vi "Unflatten Packet Header.vi"(8 "error in (no error)":errorcluster, 10 "Bytes in":u8[](array[numeric]), 11 "pcap Parse and Build in":refnum<class "pcap Parse and Build.lvclass">) -> (0 "error out":errorcluster, 1 "Packet Header":T1, 2 "Bytes out":u8[](array[numeric]), 3 "pcap Parse and Build out":refnum<class "pcap Parse and Build.lvclass">)   [LabVIEW 2021, in "pcap Parse and Build.lvclass"]
uses:
  pcap Parse and Build.lvclass
  Typedef/Packet Header.ctl
  pcap Parse and Build.lvclass/pcap Parse and Build.ctl
  Typedef/Errors.ctl
  a43927ee-7cb0-4c47-8c72-c2f3daaaf6fd.vi
  a43927ee-7cb0-4c47-8c72-c2f3daaaf6fd.vi/c28b0ead-42ad-4072-80a2-aca7f2bd7ce3.vi
  <vilib>/CIF Foundation/CIF Utilities/Errors/Append Error Location.vi
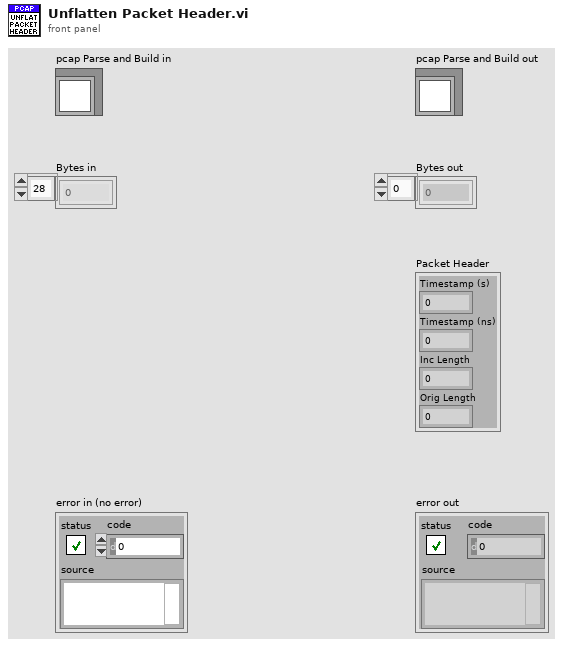
[diagram p1: front panel]
types:
  T1 = typedef "pcap Parse and Build.lvclass/Packet Header.ctl" = cluster{"Timestamp (s)":u32, "Timestamp (ns)":u32, "Inc Length":u32, "Orig Length":u32}
  T2 = typedef "pcap Parse and Build.lvclass/Errors.ctl" = enum16{"Invalid Global Header", "Out of Data"}
  T3 = typedef "pcap Parse and Build.lvclass/Time Format.ctl" = enum16{"us", "ns"}
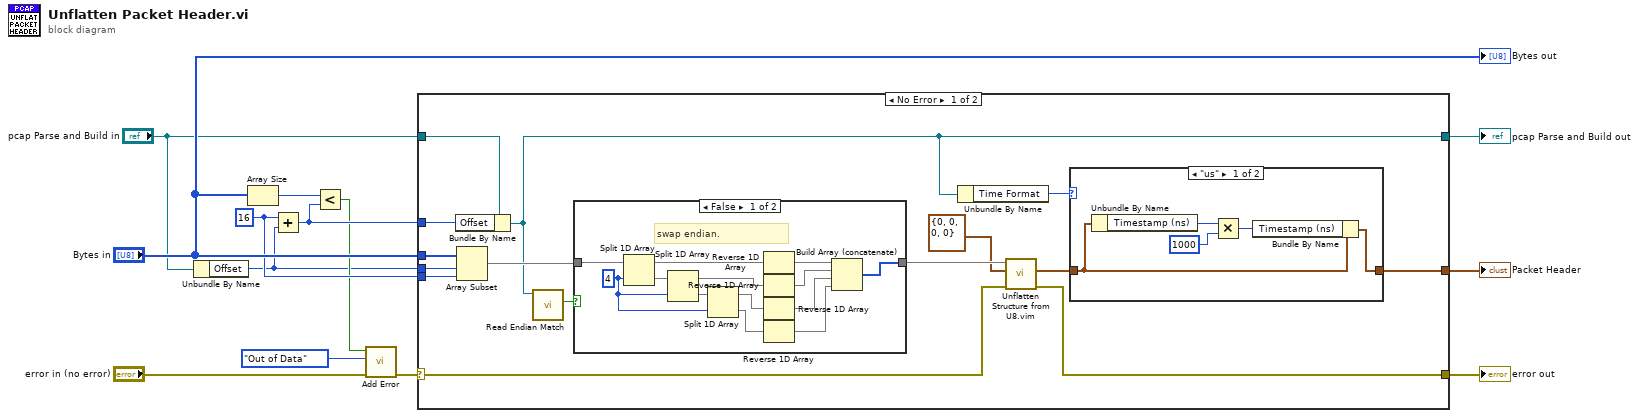
[diagram p0: block diagram]
diagram:
  w10 = 16 ("length")
  n1 = Unbundle By Name("pcap Parse and Build in") -> ("Offset"=w3:i32)
  n2 = Array Size(array="Bytes in") -> (size(s)=w5:i32)
  n3 = Add(x=w10, y=w3) -> (x+y=w11:i32)
  n4 = Less?(x=w5, y=w11) -> (x < y?=w9:bool)
  n5 = call "Add Error.vi"("error in (no error)"="error in (no error)", "Error"=Errors."Out of Data", "Insert Error"=w9) -> ("error out"=w6:errorcluster)  [unwired: 8 in]
  n6 = case shown="No Error" w6 {
    selector: w6 -> [w27 w50]
    tunnel: [w28 w50] -> w4
    tunnel: [w23 _] -> w13
    tunnel: "Bytes in" -> [w25 _]
    tunnel: w11 -> [w19 _]
    tunnel: w10 -> [w22 _]
    tunnel: w3 -> [w21 _]
    tunnel: "pcap Parse and Build in" -> [w20 w49]
    tunnel: [w17 w49] -> w1
    frame No Error {
      n7 = Bundle By Name(cluster=w20, "Offset"=w19) -> (w17:refnum<class "pcap Parse and Build.lvclass">)
      n8 = Array Subset(array=w25, index=w21, length=w22) -> (w24:u8[])
      n9 = call "Read Endian Match.vi"("pcap Parse and Build in"=w17) -> ("Endian Match"=w18:bool)  [unwired: 8 in, 2 out]
      n10 = case shown="False" w18 {
        tunnel: w24 -> [w34 w42]
        tunnel: [w29 w42] -> w26
        frame False {
          w39 = 4 ("index")
          # "swap endian."
          n11 = Split 1D Array(array=w34, index=w39) -> (first subarray=w37:u8[], second subarray=w41:u8[])
          n12 = Split 1D Array(array=w41, index=w39) -> (first subarray=w36:u8[], second subarray=w40:u8[])
          n13 = Split 1D Array(array=w40, index=w39) -> (first subarray=w35:u8[], second subarray=w38:u8[])
          n14 = Reverse 1D Array(array=w37) -> (reversed array=w33:u8[])
          n15 = Reverse 1D Array(array=w36) -> (reversed array=w32:u8[])
          n16 = Reverse 1D Array(array=w35) -> (reversed array=w31:u8[])
          n17 = Reverse 1D Array(array=w38) -> (reversed array=w30:u8[])
          n18 = Build Array (concatenate)(w33, w32, w31, w30) -> (w29:u8[])
        }
        frame True {
        }
      }
      n19 = Unbundle By Name(w17) -> ("Time Format"=w16:T3)
      n20 = call "Unflatten Structure from U8.vim"("error in"=w27, "Type"=T1 {"Timestamp (s)"=0, "Timestamp (ns)"=0, "Inc Length"=0, "Orig Length"=0}, "Flattend Data in"=w26) -> ("error out"=w28:errorcluster, "Unflattend Data"=w14:T1)  [unwired: 6 in, 1 out]
      n21 = case shown="\"us\"" w16 {
        tunnel: w14 -> [w43 w48]
        tunnel: [w44 w48] -> w23
        frame "us" {
          n22 = Unbundle By Name(w43) -> ("Timestamp (ns)"=w47:u32)
          n23 = Multiply(x=w47, y=u32 1000) -> (x*y=w45:u32)
          n24 = Bundle By Name(cluster=w43, "Timestamp (ns)"=w45) -> (w44:T1)
        }
        frame "ns", Default {
        }
      }
    }
    frame Error {
    }
  }
  "error out" <- w4
  "pcap Parse and Build out" <- w1
  "Packet Header" <- w13
  "Bytes out" <- "Bytes in"
